vi "Player Info.vi"(11 "64 in":refnum<class "64.lvclass">) -> (0 "Defeat Speech":string, 1 "Victory Speech":string, 2 "Name":string, 3 "64 out":refnum<class "64.lvclass">)   [LabVIEW 2015, in "64.lvclass"]
uses:
  64.lvclass
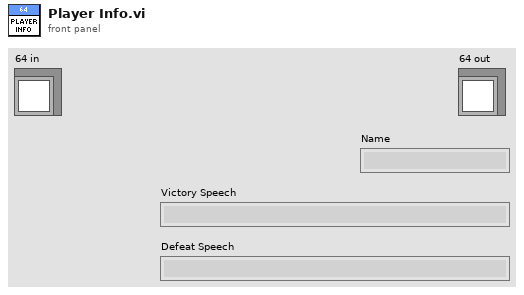
[diagram p1: front panel]
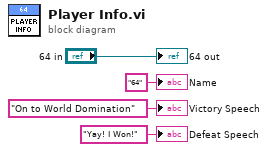
[diagram p0: block diagram]
diagram:
  "64 out" <- "64 in"
  "Name" <- "64" ("Name")
  "Victory Speech" <- "On to World Domination" ("Victory Speech")
  "Defeat Speech" <- "Yay! I Won!" ("Defeat Speech")
